vi "Update Gate Parameters Visibility.vi"(7 "Edit User-defined Gate":refnum<vi>, 10 "error in (no error)":errorcluster, 11 "Phasor Explorer Gate Parameters in":refnum<vi>) -> (2 "error out":errorcluster, 3 "Phasor Explorer Gate Parameters out":refnum<vi>)   [LabVIEW 2019]
uses:
  Phasor Explorer Gate Parameters.ctl
  Gate Type.ctl
panel:
  in  "Type of User-defined Function":enum32{"Gate", "IRF"}(radio)
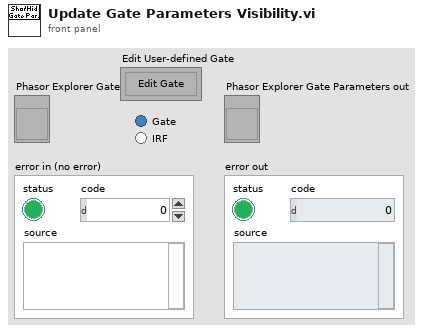
[diagram p1: front panel]
types:
  T1 = typedef "Phasor Explorer Gate Parameters.ctl" = cluster{"First Gate Start":dbl[unit], "Use Gate Center":bool, "Gate Width":dbl[unit], "Gate Step":dbl[unit], "# Gates":dbl, "Gate Type":T2, "Edge Width":dbl[unit], "Top Slope":dbl[unit], "Reversed Sawtooth?":bool, "Analytical Computation":bool, "Tolerance":dbl, "Integration":enum32{"Item 0", "Item 1"}, "# Steps":dbl, "Type of User-defined Function":enum32{"Gate", "IRF"}}
  T2 = typedef "Gate Type.ctl" = enum16{"Square", "Finite Edge Square", "Finite Edge, Tilted Top Square", "Triangle", "Sawtooth", "User-defined"}
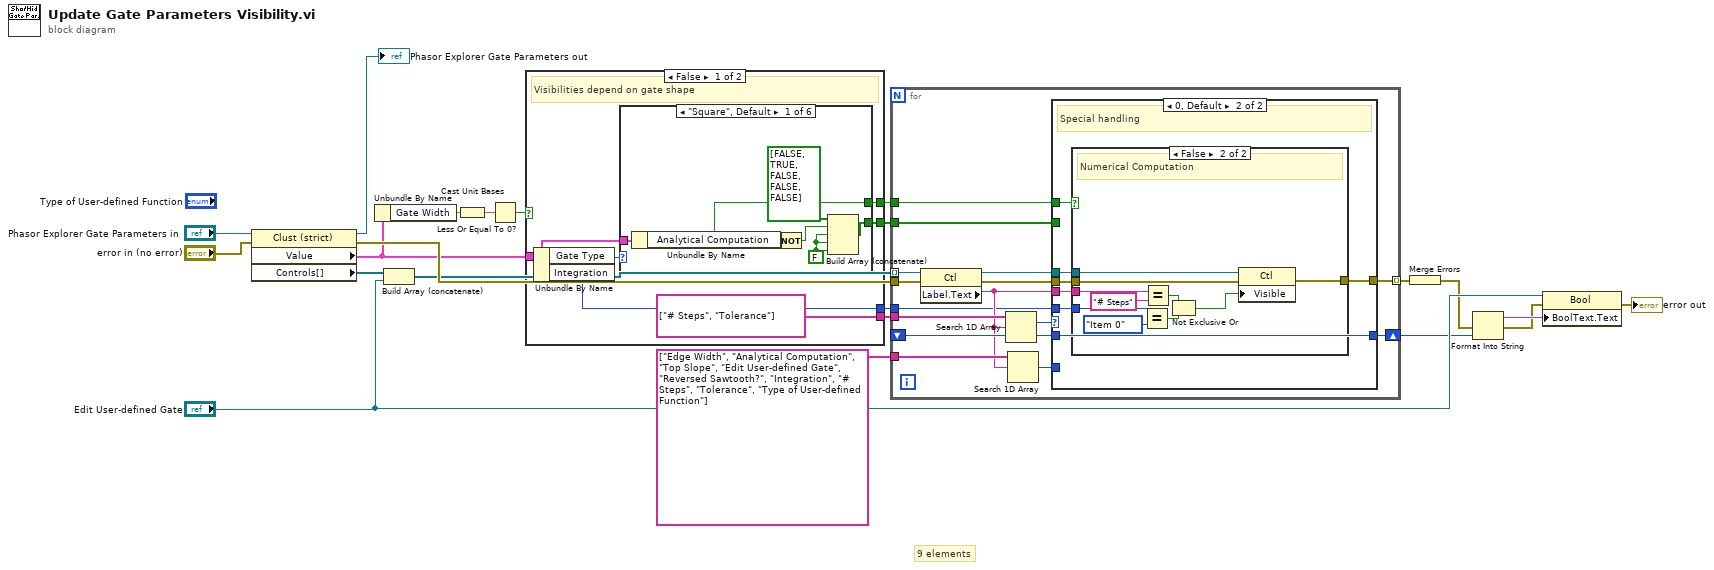
[diagram p0: block diagram]
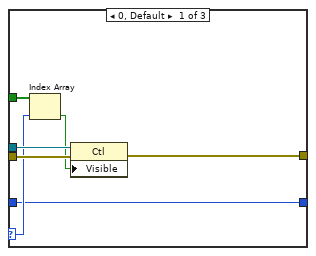
[diagram p3: hidden frame]
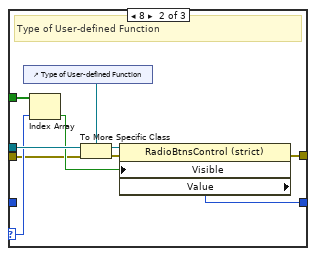
[diagram p4: hidden frame]
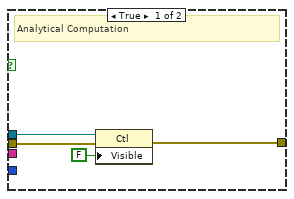
[diagram p5: hidden frame]
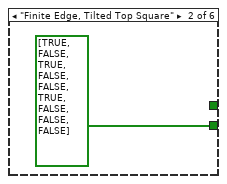
[diagram p6: hidden frame]
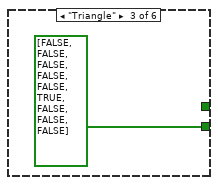
[diagram p7: hidden frame]
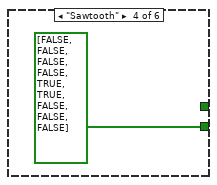
[diagram p8: hidden frame]
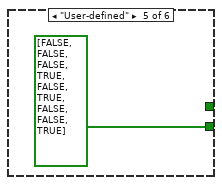
[diagram p9: hidden frame]
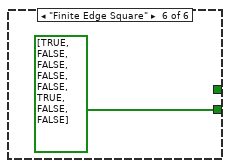
[diagram p10: hidden frame]
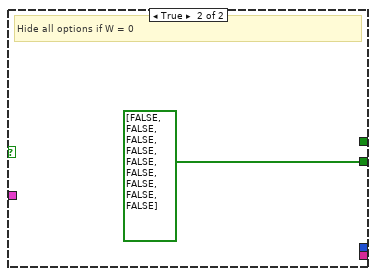
[diagram p11: hidden frame]
diagram:
  # "9 elements"
  n1 = property class="Clust (strict)"(reference="Phasor Explorer Gate Parameters in", error in="error in (no error)") -> (reference out=→"Phasor Explorer Gate Parameters out":refnum<vi>, error out=w17:errorcluster, "Value"=w14:T1, "Controls[]"=w18:refnum<vi>[])
  n2 = Unbundle By Name(w14) -> ("Gate Width"=w13:dbl[unit])
  n3 = Build Array (concatenate)(w18, "Edit User-defined Gate") -> (w10:refnum<vi>[])
  n4 = Cast Unit Bases(0:w13) -> (2:w12:dbl)  [unwired: 1 in]
  n5 = Less Or Equal To 0?(x=w12) -> (x <= 0?=w11:bool)
  n6 = case shown="False" w11 {
    tunnel: w14 -> [w27 _]
    tunnel: [w26 bool[] [FALSE, FALSE, FALSE, FALSE, FALSE, FALSE, FALSE, FALSE, FALSE] ("Label.Text")] -> w16
    tunnel: [w25 _] -> w9
    tunnel: [string[] ["# Steps", "Tolerance"] ("Label.Text") _] -> w2
    tunnel: [w23 _] -> w1
    frame False {
      # "Visibilities depend on gate shape"
      n7 = Unbundle By Name(w27) -> ("Gate Type"=w28:T2, "Integration"=w23:enum32{"Item 0", "Item 1"})
      n8 = case shown="\"Square\", Default" w28 {
        tunnel: w27 -> [w34 _ _ _ _ _]
        tunnel: [w32 bool[] [TRUE, FALSE, TRUE, FALSE, FALSE, TRUE, FALSE, FALSE, FALSE] ("Label.Text") bool[] [FALSE, FALSE, FALSE, FALSE, FALSE, TRUE, FALSE, FALSE, FALSE] ("Label.Text") bool[] [FALSE, FALSE, FALSE, FALSE, TRUE, TRUE, FALSE, FALSE, FALSE] ("Label.Text") bool[] [FALSE, FALSE, FALSE, TRUE, FALSE, TRUE, FALSE, FALSE, TRUE] ("Label.Text") bool[] [TRUE, FALSE, FALSE, FALSE, FALSE, TRUE, FALSE, FALSE] ("Label.Text")] -> w26
        tunnel: [w30 _ _ _ _ _] -> w25
        frame "Square", Default {
          w29 = FALSE ("element")
          n9 = Unbundle By Name(w34) -> ("Analytical Computation"=w30:bool)
          n10 = Not(x=w30) -> (.not. x?=w31:bool)
          n11 = Build Array (concatenate)(bool[] [FALSE, TRUE, FALSE, FALSE, FALSE] ("Label.Text"), w31, w29, w29, w29) -> (w32:bool[])
        }
        frame "Finite Edge, Tilted Top Square" {
        }
        frame "Triangle" {
        }
        frame "Sawtooth" {
        }
        frame "User-defined" {
        }
        frame "Finite Edge Square" {
        }
      }
    }
    frame True {
      # "Hide all options if W = 0"
    }
  }
  n12 = for {
    tunnel: string[] ["Edge Width", "Analytical Computation", "Top Slope", "Edit User-defined Gate", "Reversed Sawtooth?", "Integration", "# Steps", "Tolerance", "Type of User-defined Function"] ("Label.Text") -> [w55]
    tunnel: w10 -> [w54] mode=indexing
    tunnel: w17 -> [w53]
    tunnel: w16 -> [w52]
    tunnel: [w50] -> w15 mode=indexing
    tunnel: w9 -> [w47]
    shift-right: [w46] -> w6
    shift-left: _ -> [w45]
    tunnel: w2 -> [w43]
    tunnel: w1 -> [w41]
    n13 = property class="Ctl"(reference=w54, error in=w53) -> (reference out=w49:refnum<vi>, error out=w48:errorcluster, "Label.Text"=w42:string)
    n14 = Search 1D Array(1D array=w43, element=w42) -> (index of element=w44:i32)  [unwired: 1 in]
    n15 = Search 1D Array(1D array=w55, element=w42) -> (index of element=w51:i32)  [unwired: 1 in]
    n16 = case shown="0, Default" w44 {
      tunnel: w52 -> [w62 _]
      tunnel: w51 -> [w61 _]
      tunnel: [w60 w88] -> w50
      tunnel: w49 -> [w59 w87]
      tunnel: w48 -> [w58 w86]
      tunnel: w47 -> [_ w84]
      tunnel: [w57 w85] -> w46
      tunnel: w45 -> [w56 w85]
      tunnel: w42 -> [_ w83]
      tunnel: w41 -> [_ w82]
      frame -1 {
        n17 = case shown="-1" w61 {
          selector: w61 -> [w66 w77 _]
          tunnel: w59 -> [w69 w79 _]
          tunnel: w58 -> [w68 w73 w81]
          tunnel: w62 -> [w67 w78 _]
          tunnel: [w64 w75 w81] -> w60
          tunnel: [w63 w70 w80] -> w57
          tunnel: w56 -> [w63 _ w80]
          frame 0, Default {
            n18 = Index Array(array=w67, index=w66) -> (element=w65:bool)
            n19 = property class="Ctl"(reference=w69, error in=w68, "Visible"=w65) -> (error out=w64:errorcluster)  [unwired: 1 out]
          }
          frame 8 {
            # "Type of User-defined Function"
            n20 = control-ref of="Type of User-defined Function"() -> (w71:refnum<vi>)
            n21 = Index Array(array=w78, index=w77) -> (element=w76:bool)
            n22 = To More Specific Class(target class=w71, reference=w79, error in=w73) -> (specific class reference=w74:refnum<vi>, error out=w72:errorcluster)
            n23 = property class="RadioBtnsControl (strict)"(reference=w74, error in=w72, "Visible"=w76) -> (error out=w75:errorcluster, "Value"=w70:enum32{"Gate", "IRF"})  [unwired: 1 out]
          }
          frame -1 {
          }
        }
      }
      frame 0, Default {
        # "Special handling"
        n24 = case shown="False" w84 {
          tunnel: [w92 w102] -> w88
          tunnel: w87 -> [w91 w101]
          tunnel: w86 -> [w90 w100]
          tunnel: w83 -> [_ w97]
          tunnel: w82 -> [_ w99]
          frame True {
            # "Analytical Computation"
            n25 = property class="Ctl"(reference=w91, error in=w90, "Visible"=FALSE) -> (error out=w92:errorcluster)  [unwired: 1 out]
          }
          frame False {
            # "Numerical Computation"
            n26 = Equal?(x=w99, y=enum32{"Item 0", "Item 1"}."Item 0" ("Integration")) -> (x = y?=w94:bool)
            n27 = Equal?(x=w97, y="# Steps" ("Label.Text")) -> (x = y?=w95:bool)
            n28 = Not Exclusive Or(1:w94, 2:w95) -> (0:w93:bool)
            n29 = property class="Ctl"(reference=w101, error in=w100, "Visible"=w93) -> (error out=w102:errorcluster)  [unwired: 1 out]
          }
        }
      }
    }
  }
  n30 = Merge Errors(w15) -> (w4:errorcluster)
  n31 = Format Into String(error in=w4, w6) -> (resulting string=w5:string, error out=w3:errorcluster)  [unwired: 2 in]
  n32 = property class="Bool"(reference="Edit User-defined Gate", error in=w3, "BoolText.Text"=w5) -> (error out=→"error out":errorcluster)  [unwired: 1 out]
